vi "create subfolder.vi"(8 "error in (no error)":errorcluster, 10 "Folder Name":string, 11 "FolderPath":path) -> (0 "error out":errorcluster, 3 "Subfolder path":path)   [LabVIEW 2012, in "Design Server.lvlib"]
uses:
  Design Server.lvlib
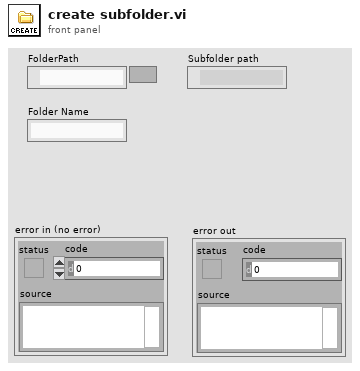
[diagram p1: front panel]
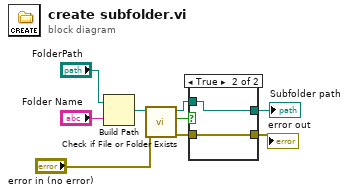
[diagram p0: block diagram]
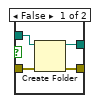
[diagram p2: hidden frame]
diagram:
  n1 = Build Path(base path="FolderPath", name or relative path="Folder Name") -> (appended path=w5:path)
  n2 = call <vilib>:"Check if File or Folder Exists.vi"("error in (no error)"="error in (no error)", "path"=w5) -> ("error out"=w8:errorcluster, "file or folder exists?"=w6:bool, "dup path"=w7:path)  [unwired: 7 in]
  n3 = case shown="True" w6 {
    tunnel: w7 -> [w13 w15]
    tunnel: w8 -> [w12 w14]
    tunnel: [w11 w15] -> w9
    tunnel: [w10 w14] -> w2
    frame False {
      n4 = Create Folder(path (use dialog)=w13, error in=w12) -> (created path=w11:path, error out=w10:errorcluster)  [unwired: 1 in, 1 out]
    }
    frame True {
    }
  }
  "Subfolder path" <- w9
  "error out" <- w2
